vi "Ctor.vi"(8 "error in (no error)":errorcluster, 11 "Value":dbl) -> (0 "error out":errorcluster, 3 "Test Type B out":refnum<class "Test Type B.lvclass">)   [LabVIEW 2020, in "Test Type B.lvclass"]
uses:
  Test Type B.lvclass
  Ref Data.ctl
  Test Type B.lvclass/Test Type B.ctl
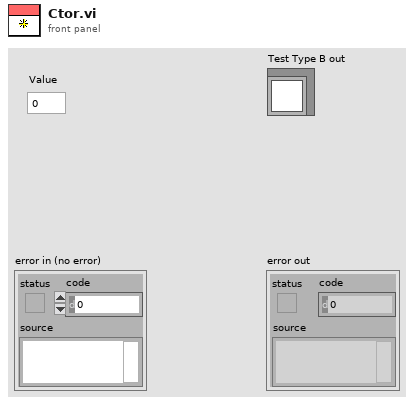
[diagram p1: front panel]
types:
  T1 = typedef "Test Type B.lvclass/Ref Data.ctl" = cluster{"Value":dbl}
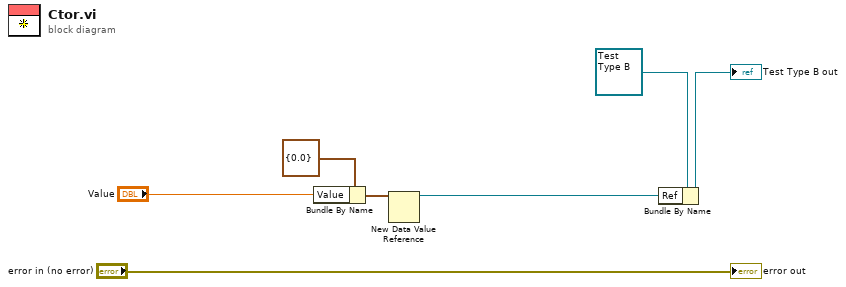
[diagram p0: block diagram]
diagram:
  n1 = Bundle By Name(cluster=T1 {"Value"=0.0} ("Ref Data"), "Value"="Value") -> (w3:T1)
  n2 = New Data Value Reference(data value=w3) -> (data value reference=w1:refnum<data-value>)  [unwired: 1 in, 1 out]
  n3 = Bundle By Name(cluster=refnum<class "Test Type B.lvclass"> refnum ("Test Type B in"), "Ref"=w1) -> (→"Test Type B out":refnum<class "Test Type B.lvclass">)
  "error out" <- "error in (no error)"
